vi "Update GlobalStop.ReaderState by ID.vi"(7 "PackageID":i32, 8 "error in":errorcluster, 11 "RunState":bool) -> (0 "error out":errorcluster)   [LabVIEW 2021, in "XNET-CAN-Signal-Logger.lvlib"]
uses:
  XNET-CAN-Signal-Logger.lvlib
  Global Variables.vi
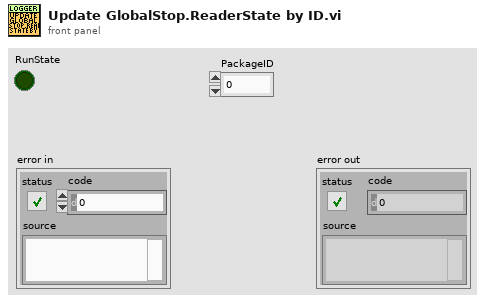
[diagram p1: front panel]
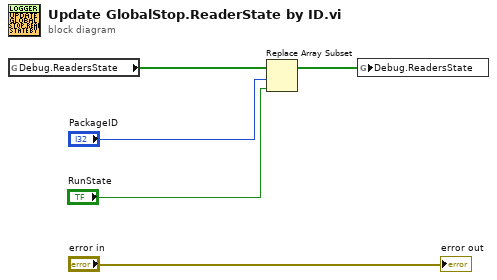
[diagram p0: block diagram]
diagram:
  n1 = global read "Global Variables.vi" "Debug.ReadersState"() -> (w1:bool[])
  n2 = Replace Array Subset(array=w1, new element="RunState", index="PackageID") -> (w4:bool[])
  n3 = global write "Global Variables.vi" "Debug.ReadersState"(w4) -> ()
  "error out" <- "error in"
